vi "IntU64ToNode(viaString).vi"(0 "Tree DVR in":refnum<data-value>, 1 "U64 in":u64, 3 "error in (no error)":errorcluster, 4 "NodePath":string) -> (5 "Tree DVR out":refnum<data-value>, 7 "error out":errorcluster)   [LabVIEW 2014]
uses:
  <vilib>/MDSplus/Classes/Tree_Class/Tree.lvclass
  <vilib>/MDSplus/Library/MDSplus.lvlib
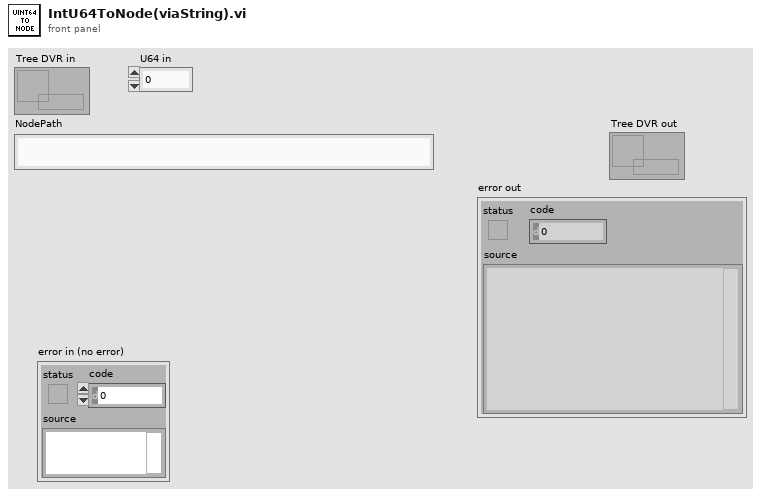
[diagram p1: front panel]
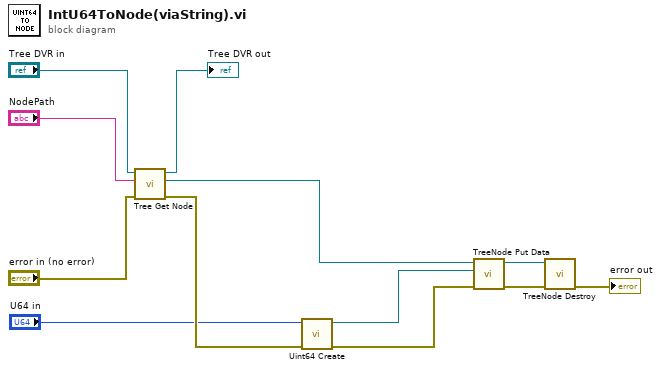
[diagram p0: block diagram]
diagram:
  n1 = call <vilib>:"Tree Get Node.vi"("error in (no error)"="error in (no error)", "Path"="NodePath", "Tree DVR in"="Tree DVR in") -> ("error out"=w10:errorcluster, "Node out"=w12:refnum<data-value>, "Tree DVR out"=→"Tree DVR out":refnum<data-value>)  [unwired: 6 in]
  n2 = call <vilib>:"Uint64 Create.vi"("error in (no error)"=w10, "U64 in"="U64 in") -> ("error out"=w11:errorcluster, "Uint64 DVR out"=w5:refnum<data-value>)  [unwired: 8 in]
  n3 = call <vilib>:"TreeNode Put Data.vi"("error in (no error)"=w11, "Data"=w5, "TreeNode DVR in"=w12) -> ("error out"=w2:errorcluster, "TreeNode DVR out"=w4:refnum<data-value>)  [unwired: 7 in]
  n4 = call <vilib>:"TreeNode Destroy.vi"("error in (no error)"=w2, "TreeNode DVR in"=w4) -> ("error out"=→"error out":errorcluster)  [unwired: 9 in]
